vi "Parameter.vi"(9 "In":string, 10 "VIId":string, 11 "VariablesRef":T3) -> ()   [LabVIEW 2018, in "Number.lvlib"]
uses:
  Number.lvlib
  <userlib>/_OpenG.lib/dictionary/dictionary.llb/Dictionary Object RefNum__ogtk.ctl
  <userlib>/_OpenG.lib/dictionary/dictionary.llb/Dictionary Object RefNum - Enum__ogtk.ctl
  <vilib>/addons/_JKI.lib/Serialization/JSON/JKI JSON Serialization.lvlib
panel:
  in  "Tab Control":enum32{"Config", "控件"}(tab)
  in  "ArrayType":T1(tab)
  in  "数值_InitialNumber":dbl caption="数值"
  in  "范围_RandomNumber":dbl=1.0 caption="范围" min=1.0
  in  "变量数量_CalculateNumber":enum16{"Single", "Double"}(ring) caption="变量数量"
  in  "公式":string
  in  "数值X_CalculateNumber":string(combo) caption="数值x"
  in  "数值Y_CalculateNumber":string(combo) caption="数值y"
  in  "数值Y_CompareNumber":string(combo) caption="数值y"
  in  "数值X_CompareNumber":string(combo) caption="数值x"
  in  "比较类型__CompareNumber":u16(ring) caption="比较类型" items=["=", "!=", ">", ">=", "<", "<="]
  in  "方法":T2(ring) caption="方法(Method)"
  # "例：x+1 或 x+y-2"
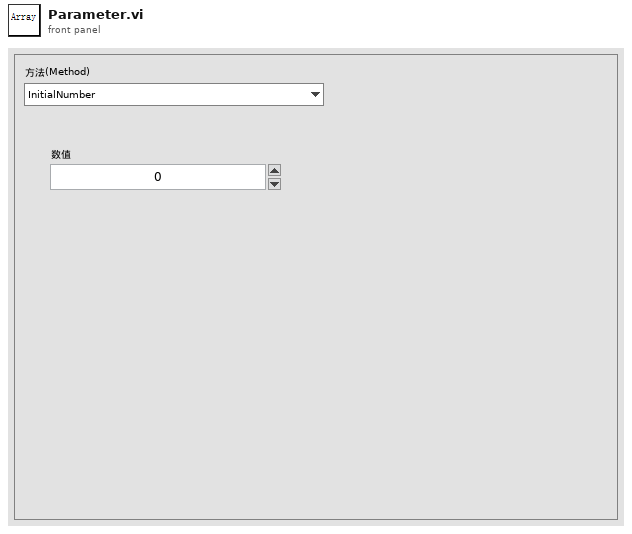
[diagram p1: front panel]
types:
  T1 = enum32{"InitialNumber", "RandomNumber", "CalculateNumber", "CompareNumber"}
  T2 = enum16{"InitialNumber", "RandomNumber", "CalculateNumber", "CompareNumber"}
  T3 = typedef "Dictionary Object RefNum__ogtk.ctl" = refnum<k1>
  T4 = cluster{"InitialNumber":cluster{"json":cluster{"Method":string, "InitialNum":dbl}}, "RandomNumber":cluster{"json":cluster{"Method":string, "Seed":dbl}}, "CalculateNumber":cluster{"json":cluster{"Method":string, "Type":string, "NumxVar":string, "NumyVar":string, "Formula":string}}, "CompareNumber":cluster{"json":cluster{"Method":string, "Type":string, "NumxVar":string, "NumyVar":string}}}
  T5 = enum32{"Invalid", "Standard", "Closed", "Hidden", "Minimized", "Maximized"}
  T6 = enum32{"invalid app kind", "Development System", "Run Time System", "Student Edition", "Embedded LabVIEW", "Evaluation", "Custom"}
  T7 = cluster{"Core":cluster{"Current VI Reference":refnum<vi>, "Close Panel on Exit?":bool}, "Parameter":cluster{"VariableRef":T3}, "Synchronize":cluster{"EnqueueData":cluster{"Action":enum16{"Create", "Query", "Revert", "UpdateVariable", "Close"}, "Data":variant}, "Echo":cluster{"VIRef":refnum<vi>, "JsonOut":string, "Status":string}, "Communicate":cluster{"ID":string, "JsonIn":string, "VarRef":T3}, "Queue":refnum<queue>}, "NumberClusters":cluster{"InitialNumber":cluster{"json":cluster{"Method":string, "InitialNum":dbl}}, "RandomNumber":cluster{"json":cluster{"Method":string, "Seed":dbl}}, "CalculateNumber":cluster{"json":cluster{"Method":string, "Type":string, "NumxVar":string, "NumyVar":string, "Formula":string}}, "CompareNumber":cluster{"json":cluster{"Method":string, "Type":string, "NumxVar":string, "NumyVar":string}}}}
  T8 = cluster{"EnqueueData":cluster{"Action":enum16{"Create", "Query", "Revert", "UpdateVariable", "Close"}, "Data":variant}, "Echo":cluster{"VIRef":refnum<vi>, "JsonOut":string, "Status":string}, "Communicate":cluster{"ID":string, "JsonIn":string, "VarRef":T3}, "Queue":refnum<queue>}
  T9 = cluster{"Current VI Reference":refnum<vi>, "Close Panel on Exit?":bool}
  T10 = cluster{"json":cluster{"Method":string, "InitialNum":dbl}}
  T11 = cluster{"json":cluster{"Method":string, "Seed":dbl}}
  T12 = cluster{"json":cluster{"Method":string, "Type":string, "NumxVar":string, "NumyVar":string, "Formula":string}}
  T13 = cluster{"json":cluster{"Method":string, "Type":string, "NumxVar":string, "NumyVar":string}}
  T14 = cluster{"Action":enum16{"Create", "Query", "Revert", "UpdateVariable", "Close"}, "Data":variant}
  T15 = cluster{"ID":string, "JsonIn":string, "VarRef":T3}
  T16 = enum16{"Create", "Query", "Revert", "UpdateVariable", "Close"}
  T17 = cluster{"VIRef":refnum<vi>, "JsonOut":string, "Status":string}
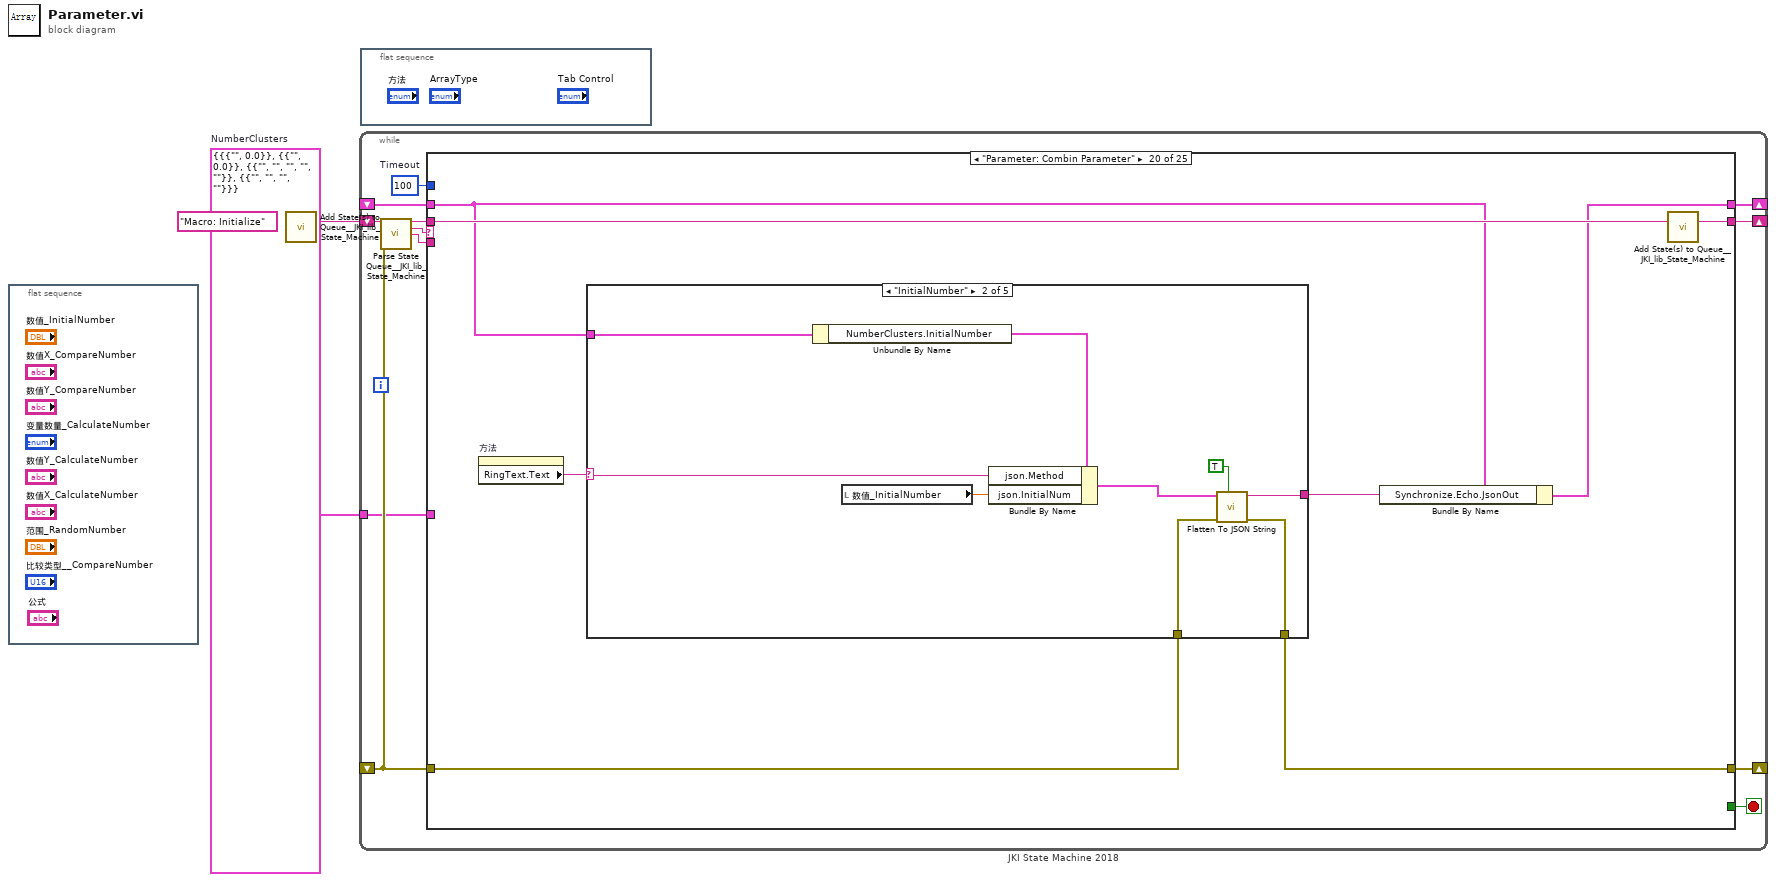
[diagram p0: block diagram]
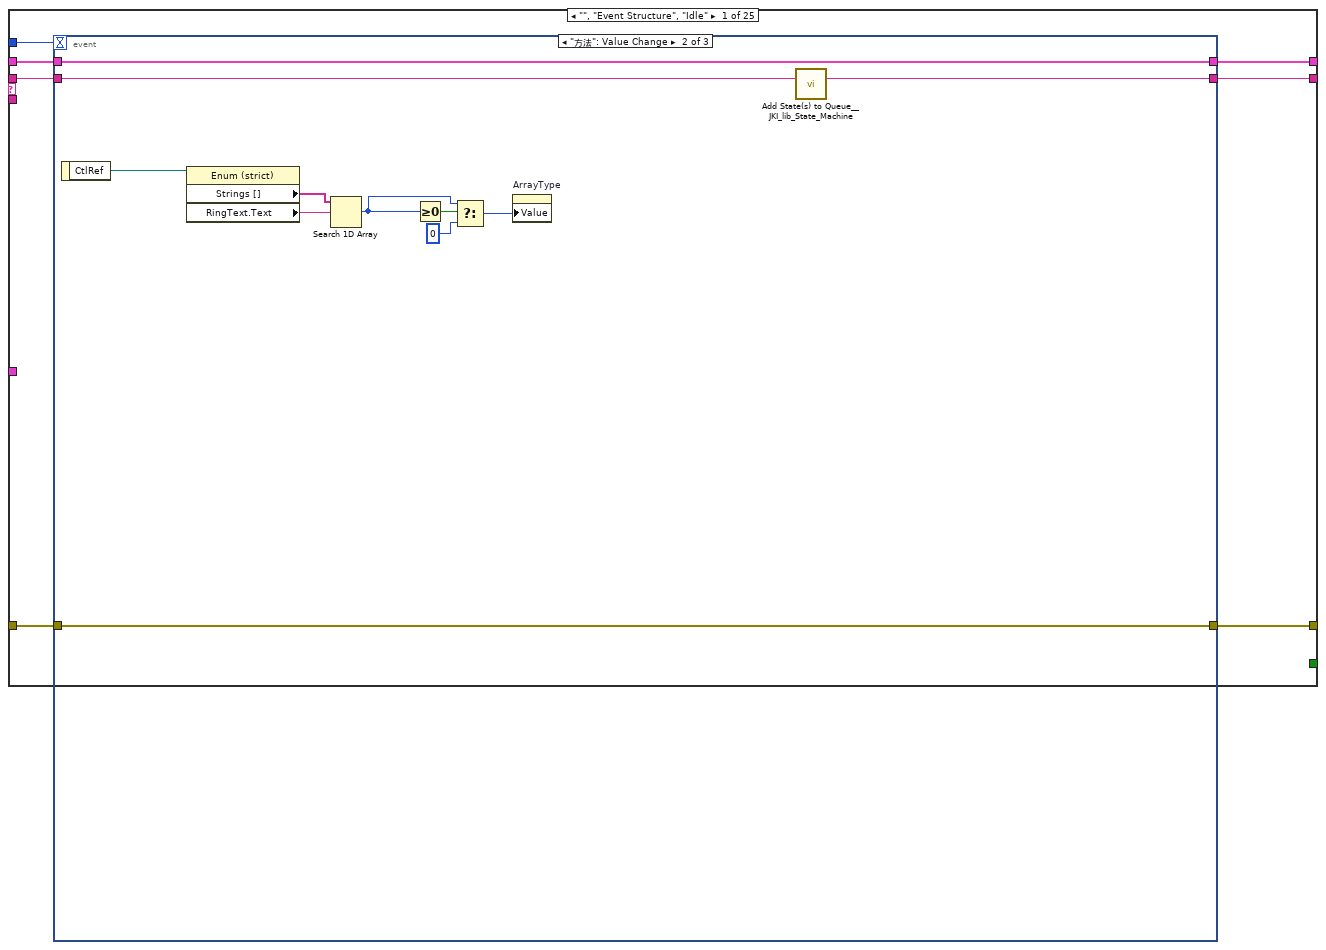
[diagram p2: hidden frame]
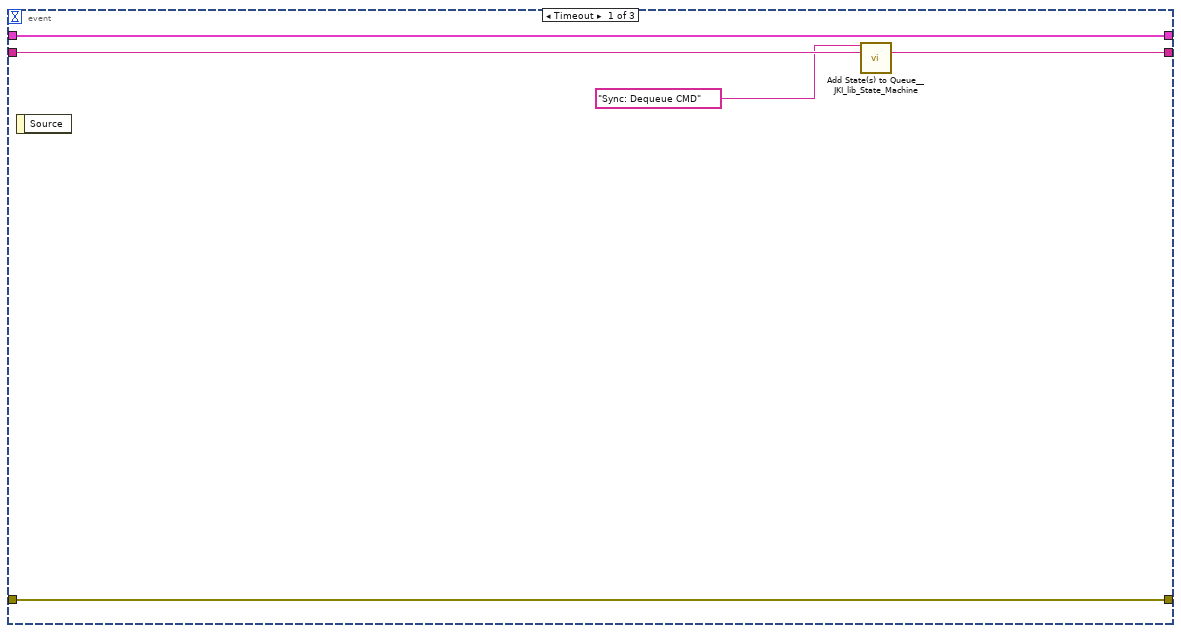
[diagram p3: hidden frame]
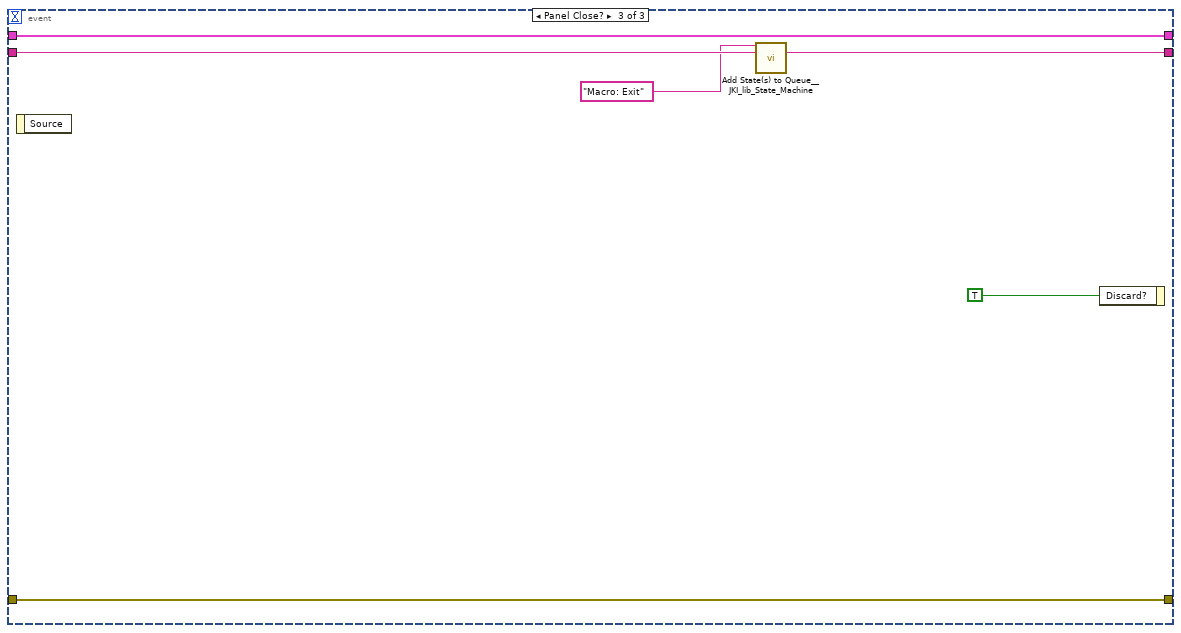
[diagram p4: hidden frame]
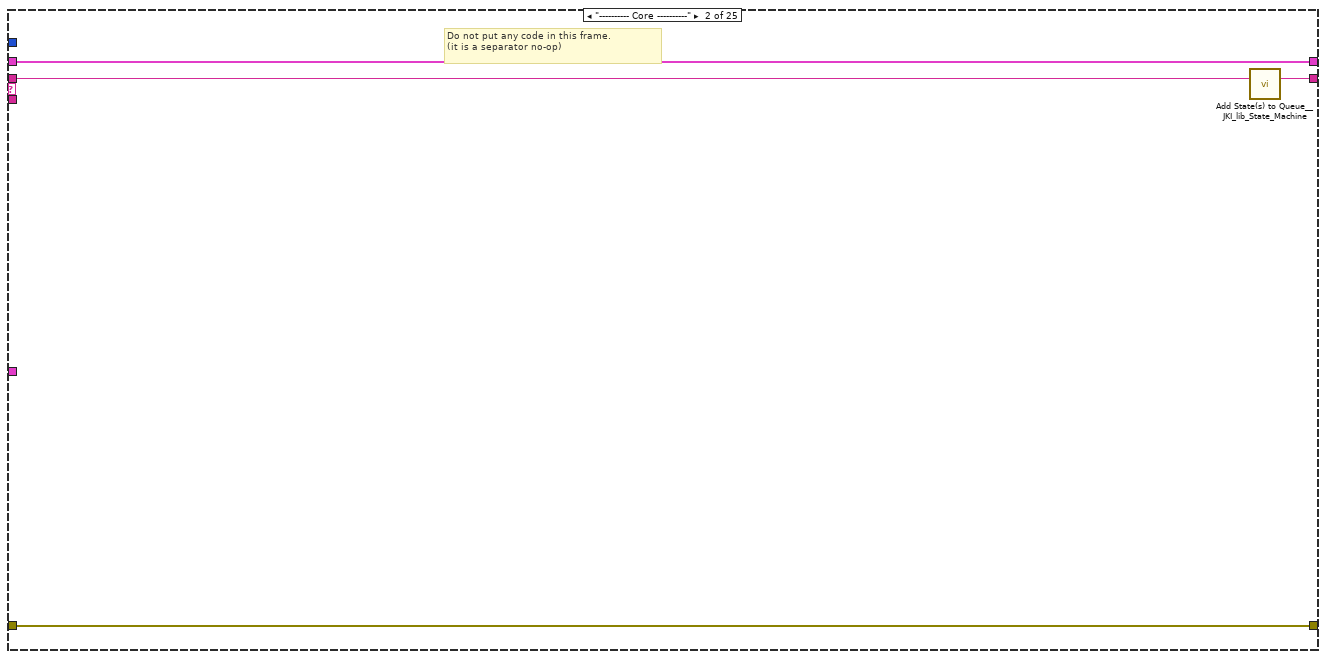
[diagram p5: hidden frame]
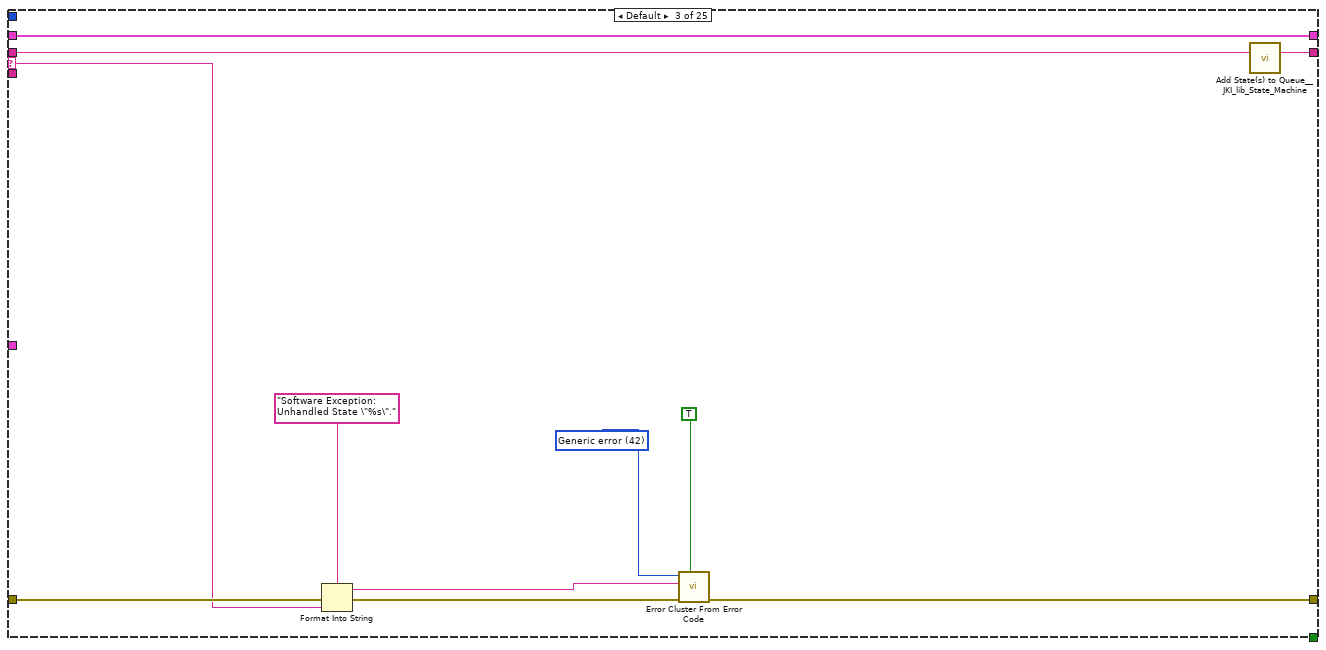
[diagram p6: hidden frame]
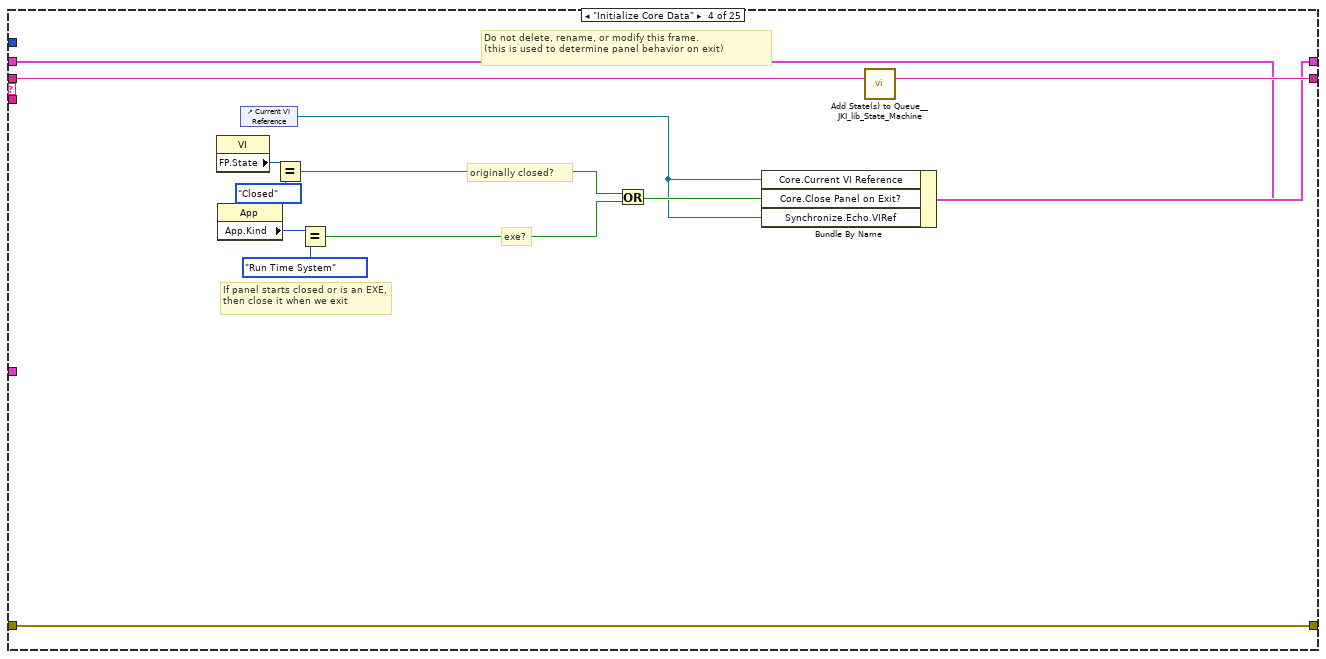
[diagram p7: hidden frame]
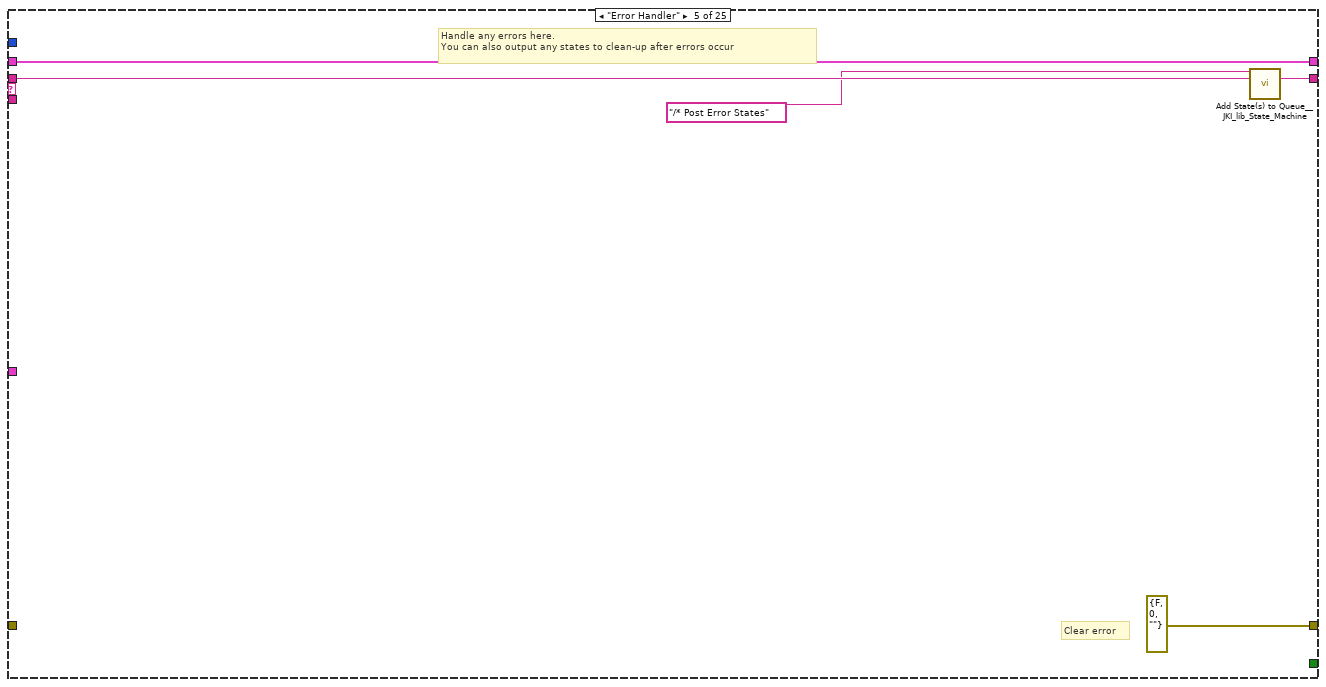
[diagram p8: hidden frame]
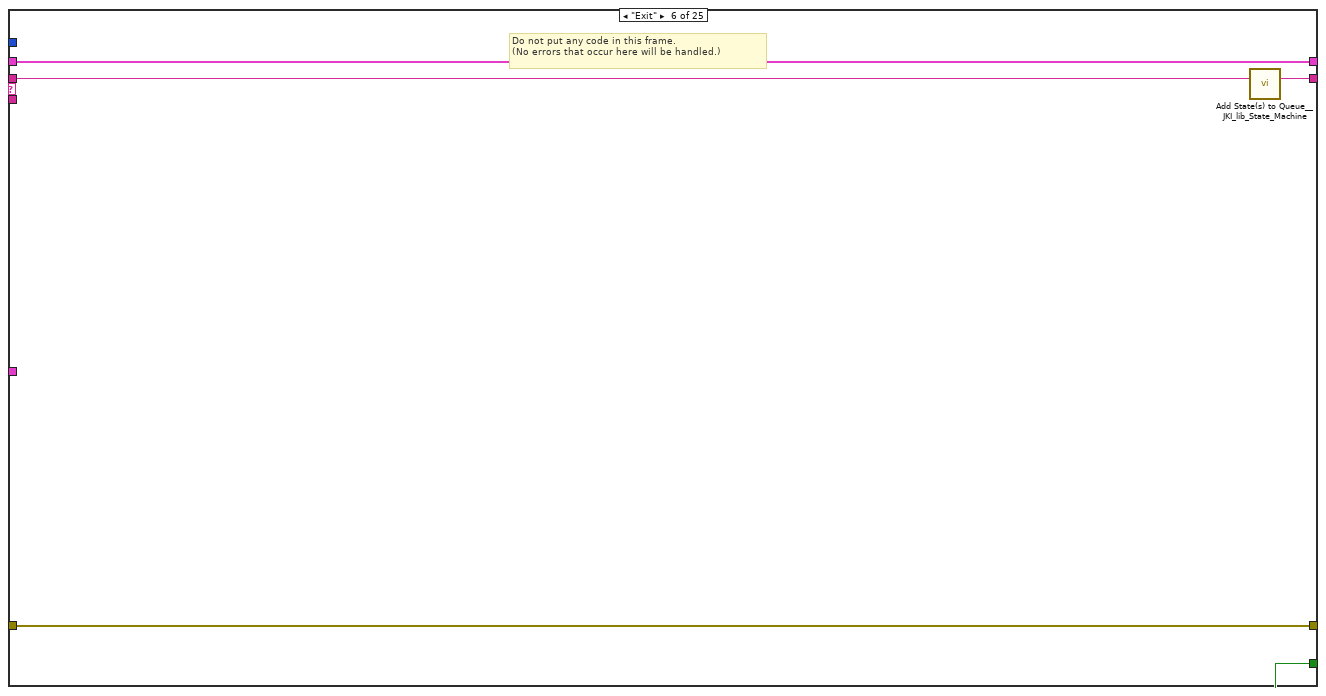
[diagram p9: hidden frame]
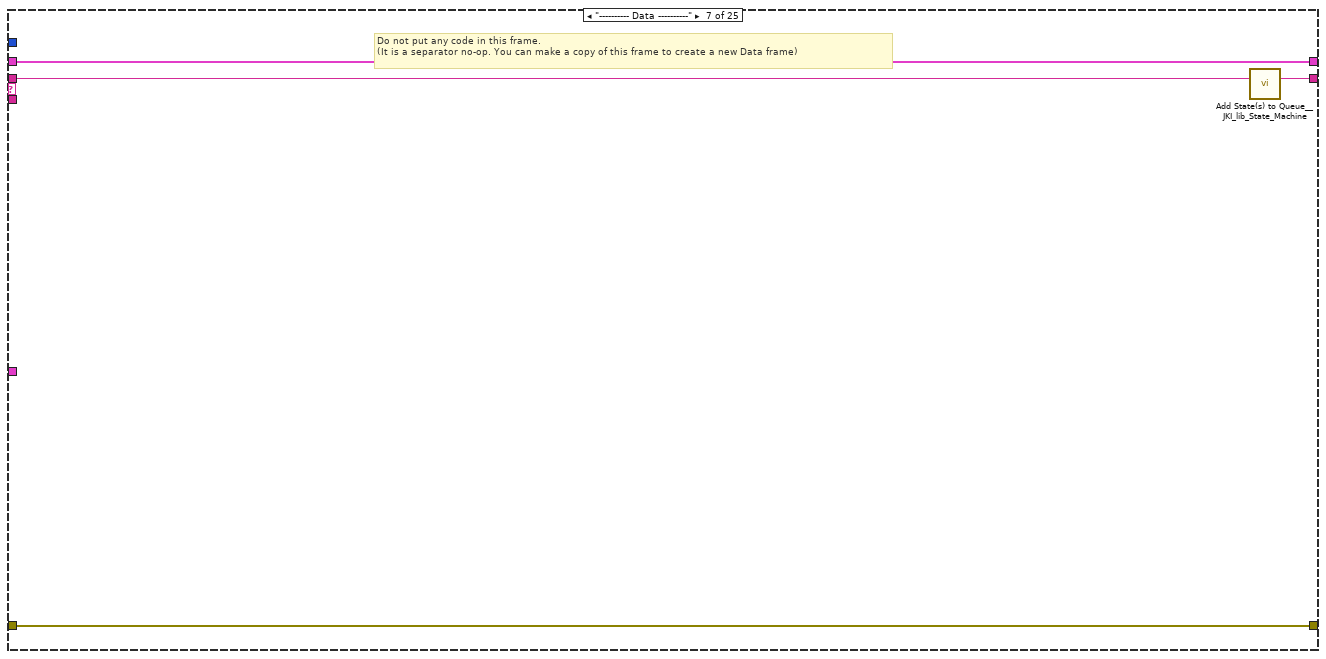
[diagram p10: hidden frame]
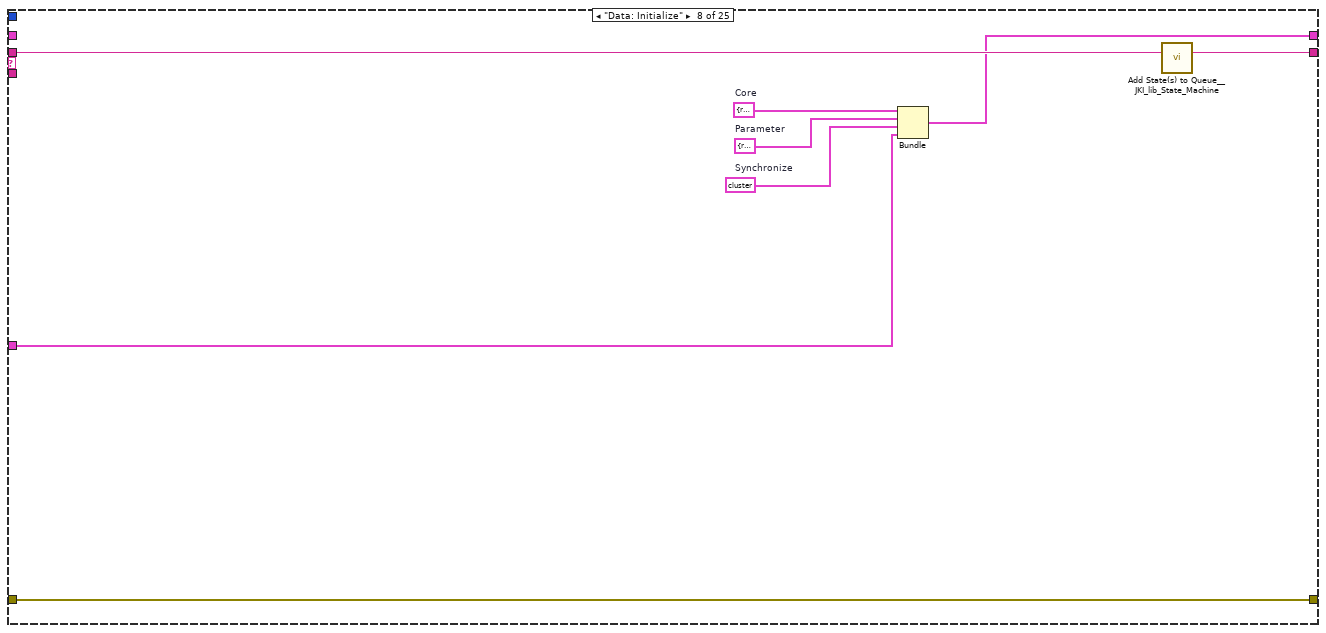
[diagram p11: hidden frame]
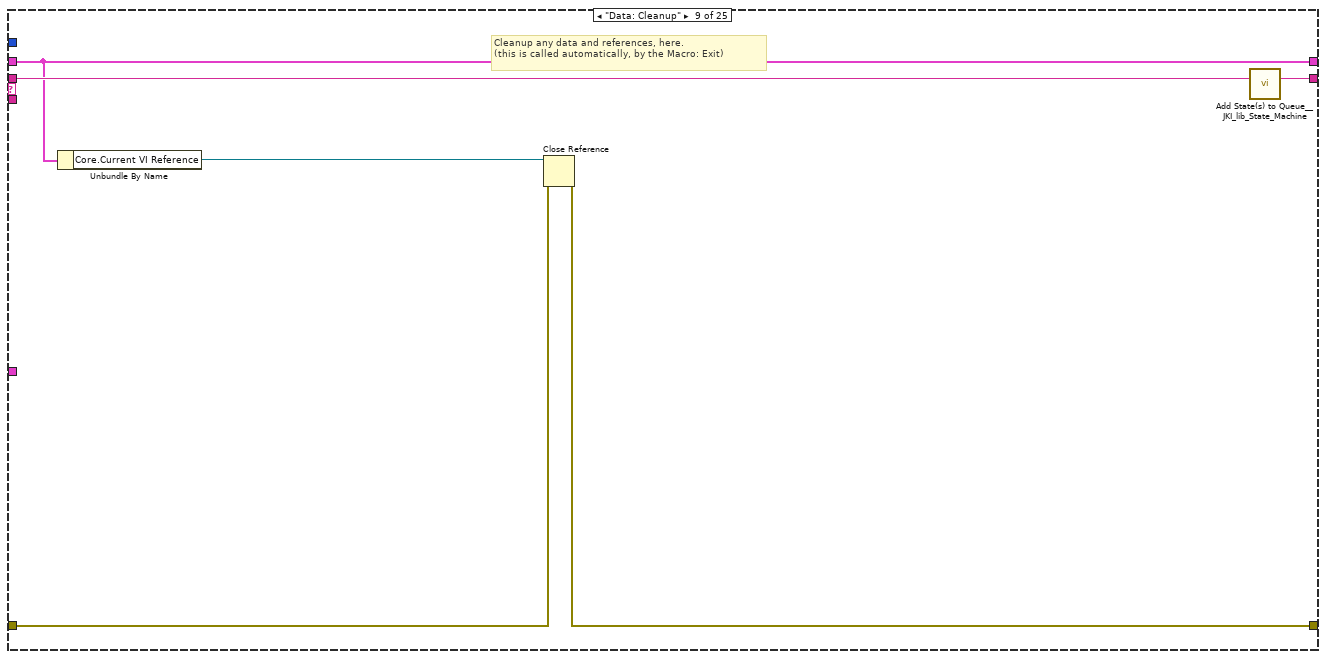
[diagram p12: hidden frame]
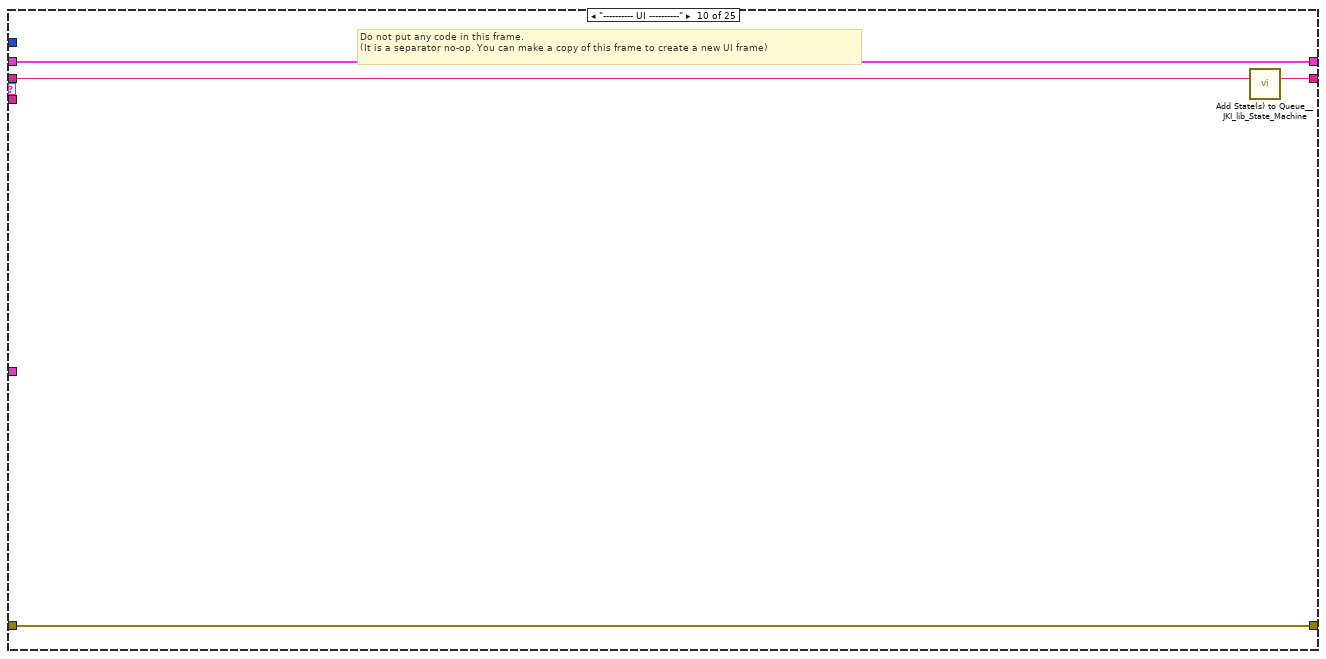
[diagram p13: hidden frame]
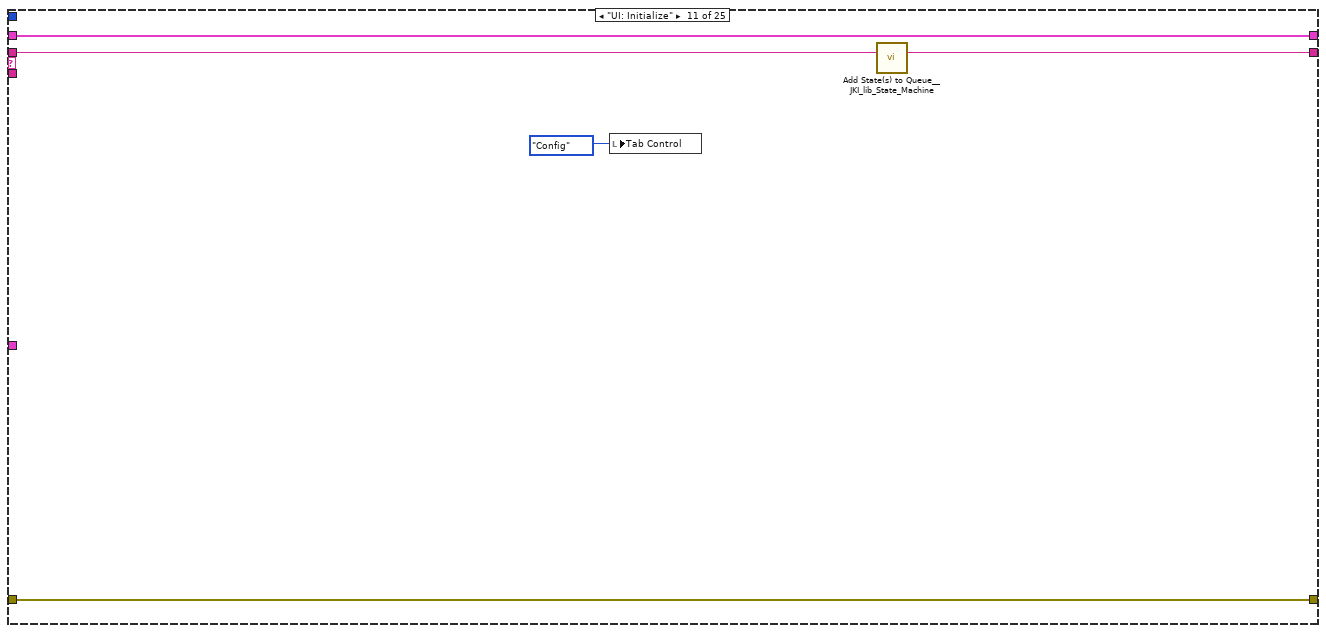
[diagram p14: hidden frame]
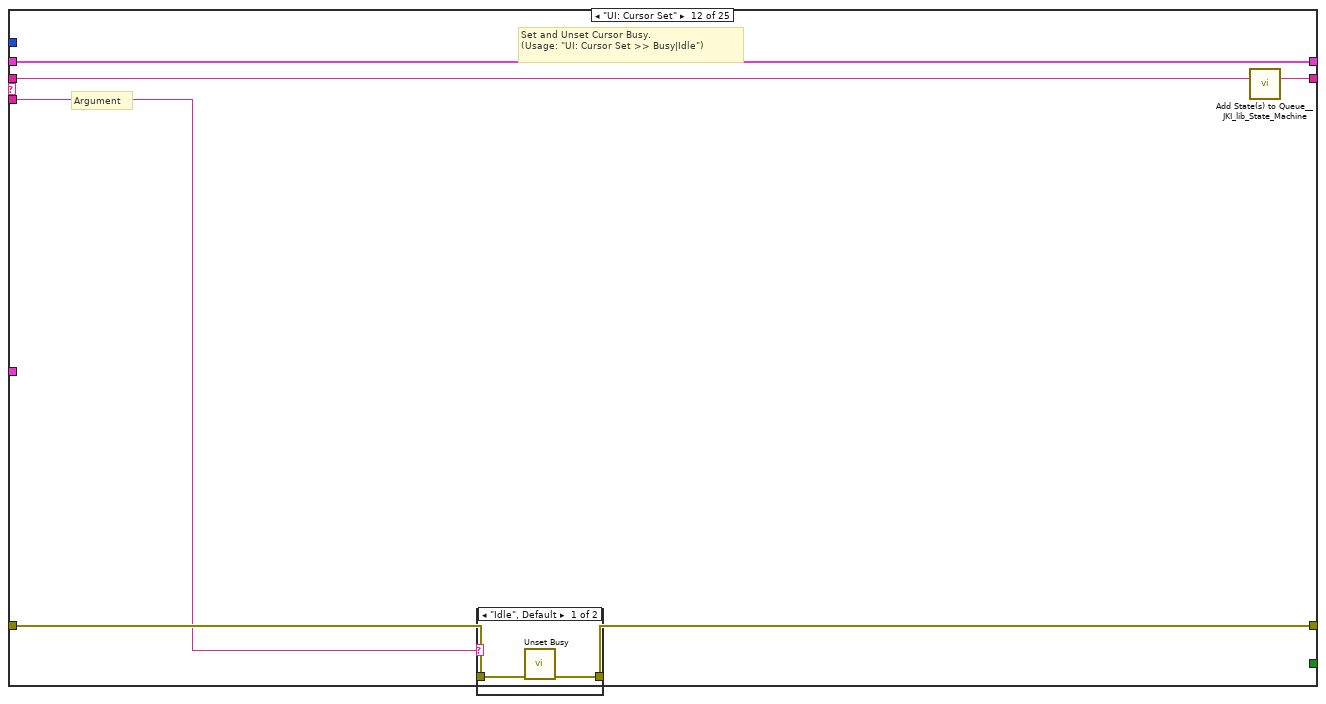
[diagram p15: hidden frame]
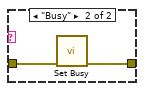
[diagram p16: hidden frame]
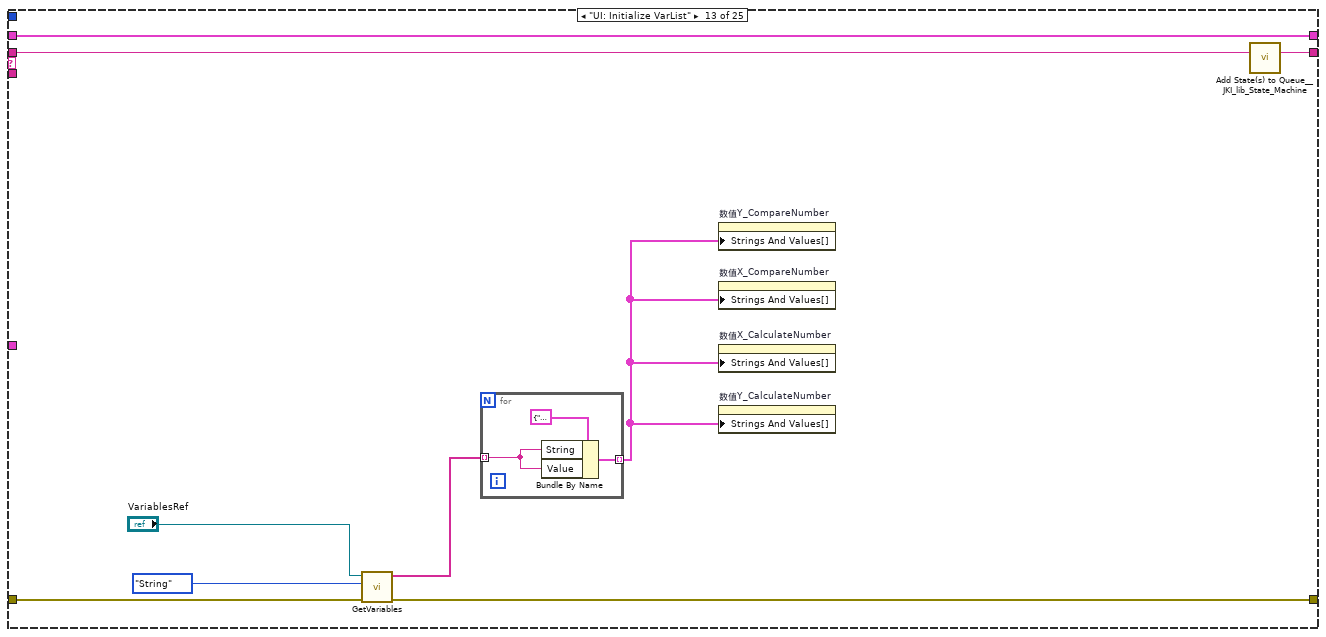
[diagram p17: hidden frame]
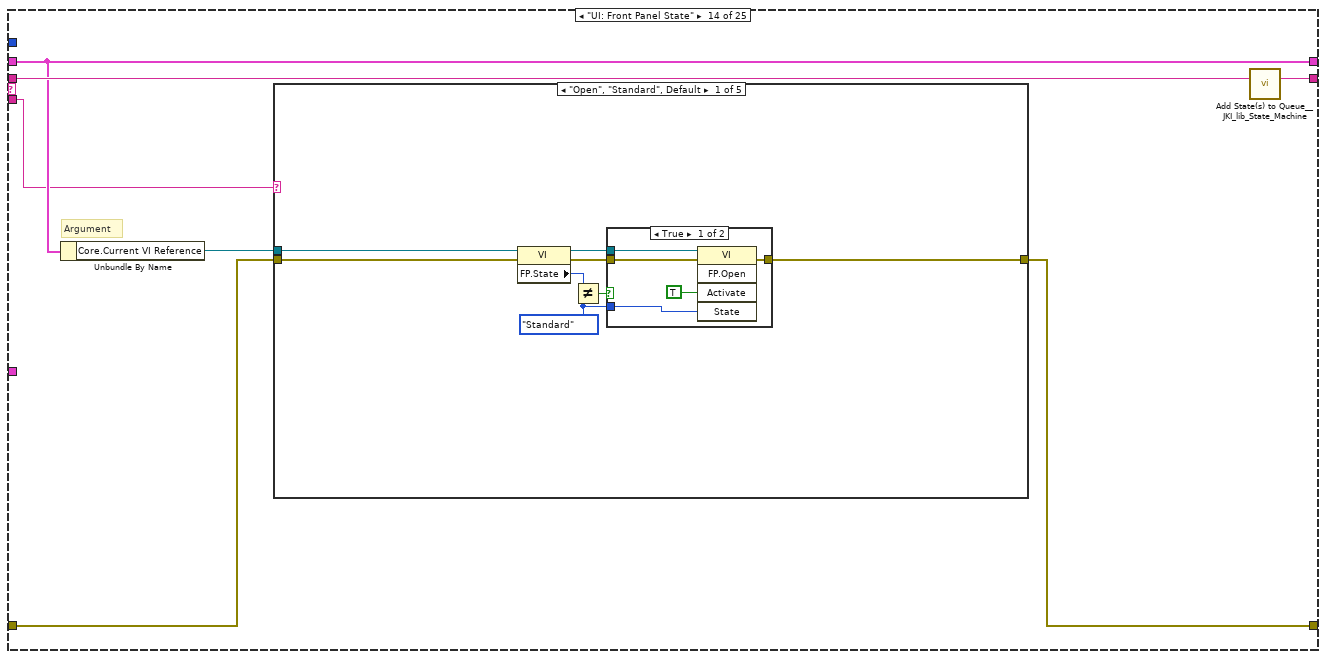
[diagram p18: hidden frame]
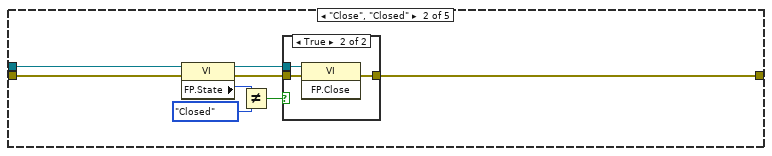
[diagram p20: hidden frame]
diagram:
  w1 = T4 {"InitialNumber"={"json"={"Method"="", "InitialNum"=0.0}}, "RandomNumber"={"json"={"Method"="", "Seed"=0.0}}, "CalculateNumber"={"json"={"Method"="", "Type"="", "NumxVar"="", "NumyVar"="", "Formula"=""}}, "CompareNumber"={"json"={"Method"="", "Type"="", "NumxVar"="", "NumyVar"=""}}}  # NumberClusters
  n1 = flat-sequence {
    frame #0 {
    }
  }
  n2 = call <vilib>:"Add State(s) to Queue__JKI_lib_State_Machine.vi"("State(s) in (\"\")"="Macro: Initialize") -> ("States Out"=w3:string)  [unwired: 14 in]
  n3 = while "JKI State Machine 2018" {
    shift-right: [w8] -> _
    shift-left: _ -> [w7]
    shift-right: [w11] -> _
    shift-left: _ -> [w5]
    shift-right: [w10] -> _
    shift-left: w3 -> [w12]
    tunnel: w1 -> [w4]
    stop <- w9 stop-if-true
    w6 = 100  # Timeout
    n4 = call <vilib>:"Parse State Queue__JKI_lib_State_Machine.vi"("State Queue"=w12, "Error In (no error)"=w5) -> ("Remaining States"=w14:string, "Current State"=w15:string, "Arguments"=w13:string)  [unwired: 11 in]
    n5 = case shown="\"Parameter: Combin Parameter\"" w15 {
      selector: w15 -> [_ _ w49 _ _ _ _ _ _ _ _ _ _ _ _ _ _ _ _ _ _ _ _ _ _]
      tunnel: w14 -> [w22 w48 w53 w72 w77 w82 w86 w94 w100 w104 w109 w115 w128 w138 w207 w212 w222 w226 w234 w313 w359 w368 w383 w427 w442]
      tunnel: w13 -> [_ _ _ _ _ _ _ _ _ _ _ w110 _ w132 _ _ _ _ _ _ _ _ _ _ _]
      tunnel: w7 -> [w20 w45 w51 w65 w74 w80 w83 _ w95 w101 w106 w113 w126 w134 w204 w209 w219 w223 w229 w310 w356 w361 w381 w424 w431]
      tunnel: [w19 w46 w55 w69 errorcluster {"status"=FALSE, "code"=0, "source"=""} ("error out") w79 w84 w92 w96 w102 w105 w111 w125 w135 w205 w210 w220 w224 w230 w309 w357 w365 w370 w422 w429] -> w11
      tunnel: w5 -> [w18 w46 w54 w69 _ w79 w84 w92 w97 w102 w105 w112 w123 w136 w205 w210 w220 w224 w231 w308 w357 w366 w379 w423 w430]
      tunnel: [w21 w47 w52 w71 w76 w81 w85 w93 w99 w103 w108 w114 w127 w137 w206 w211 w221 w225 w233 w312 w358 w367 w382 w426 w441] -> w10
      tunnel: [_ _ _ _ _ TRUE _ _ _ _ _ _ _ _ _ _ _ _ _ _ _ _ _ _ _] -> w9
      tunnel: [w17 w45 w51 w70 w74 w80 w83 w89 w95 w101 w106 w113 w126 w134 w204 w209 w219 w223 w229 w311 w356 w363 w372 w424 w431] -> w8
      tunnel: w6 -> [w16 _ _ _ _ _ _ _ _ _ _ _ _ _ _ _ _ _ _ _ _ _ _ _ _]
      tunnel: w4 -> [_ _ _ _ _ _ _ w87 _ _ _ _ _ _ _ _ _ _ _ _ _ _ _ _ _]
      frame "", "Event Structure", "Idle" {
        n6 = event shown="[1] \"方法\": Value Change" {
          selector: _ -> [_ _ _]
          dyn-events: _ -> [_ _ _]
          timeout: w16 -> [_ _ _]
          tunnel: w22 -> [w27 w38 w44]
          tunnel: [w26 w37 w43] -> w21
          tunnel: w20 -> [w24 w35 w41]
          tunnel: [w25 w36 w42] -> w19
          tunnel: w18 -> [w25 w36 w42]
          tunnel: [w24 w35 w41] -> w17
          event Timeout {
            n7 = event-data() -> ()  [unwired: 1 in, 1 out]
            n8 = call <vilib>:"Add State(s) to Queue__JKI_lib_State_Machine.vi"("State(s) in Front (\"\")"="Sync: Dequeue CMD" ("State(s) in Front (\"\")"), "State(s) in (\"\")"=w27) -> ("States Out"=w26:string)  [unwired: 13 in]
          }
          event "方法": Value Change {
            n9 = event-data() -> ("CtlRef"=w31:refnum<vi>)  [unwired: 1 in]
            n10 = property class="Enum (strict)"(reference=w31) -> ("Strings []"=w30:string[], "RingText.Text"=w29:string)  [unwired: 1 in, 2 out]
            n11 = Search 1D Array(1D array=w30, element=w29) -> (index of element=w33:i32)  [unwired: 1 in]
            n12 = Greater Or Equal To 0?(x=w33) -> (x >= 0?=w34:bool)
            n13 = Select(t=w33, s=w34, f=0) -> (s? t:f=w28:i32)
            n14 = property on="ArrayType" class="TabCtl (strict)"("Value"=w28) -> ()  [unwired: 2 in, 2 out]
            n15 = call <vilib>:"Add State(s) to Queue__JKI_lib_State_Machine.vi"("State(s) in (\"\")"=w38) -> ("States Out"=w37:string)  [unwired: 14 in]
          }
          event Panel Close? {
            n16 = event-data() -> ()  [unwired: 1 in, 1 out]
            n17 = call <vilib>:"Add State(s) to Queue__JKI_lib_State_Machine.vi"("State(s) in Front (\"\")"="Macro: Exit", "State(s) in (\"\")"=w44) -> ("States Out"=w43:string)  [unwired: 13 in]
            n18 = event-data("Discard?"=TRUE) -> ()  [unwired: 1 in, 1 out]
          }
        }
      }
      frame "---------- Core ----------" {
        # "Do not put any code in this frame.\n(it is a separator no-op)"
        n19 = call <vilib>:"Add State(s) to Queue__JKI_lib_State_Machine.vi"("State(s) in (\"\")"=w48) -> ("States Out"=w47:string)  [unwired: 14 in]
      }
      frame Default {
        w58 = 42 items=["No error", "Argument error", "Memory is full", "Out of zone", "End of file", "File already open", "Generic file I/O error", "File not found", "File permission error", "Disk is full", "Duplicate path", "Too many files open", "System feature not enabled", "Resource file not found", "Cannot add resource", "Resource not found", "Image not found", "Image memory error", "Pen does not exist", "Config type invalid", "Config token not found", "Config parse error", "Config memory error", "Bad external code format", "Bad external code offset", "External code not present", "Null window", "Destroy window error", "Null menu", "Print aborted", "Bad print record", "Print driver error", "Windows error during printing", "Memory error during printing", "Print dialog error", "Generic print error", "Invalid device refnum", "Device not found", "Device parameter error", "Device unit error", "Cannot open device", "Device call aborted", "Generic error", "Cancelled by user", "Object ID too low", "Object ID too high", "Object not in heap", "Unknown heap", "Unknown object (invalid DefProc)", "Unknown object (DefProc not in table)", "Message out of range", "Invalid (null) method", "Unknown message", "Manager call not supported", "Bad address", "Network operation in progress", "Network operation timed out", "Connection is busy", "Network attribute not supported", "Network error", "Address in use", "System out of memory", "Connection aborted", "Connection refused", "Not connected", "Already connected", "Connection closed", "Initialization error (interapplication manager)", "Bad occurrence", "Wait on unbound occurrence handler", "Occurrence queue overflow", "Datalog type conflict", "Unused", "Unrecognized type (interapplication manager)", "Memory corrupt", "Failed to make temporary DLL", "Old CIN version", "Drag socket not found", "Failed to load drop-object", "Failed to register OLE object", "Failed to release OLE object", "Format specifier type mismatch", "Unknown format specifier", "Too few format specifiers", "Too many format specifiers", "Scan failed", "Newer CIN version", "Error converting to variant", "Runtime menu error", "Password tampered", "Variant attribute not found", "Incompatible variant data type", "Event data is not available", "Event Store is not present", "Occurrence is not found", "Event Queue is not created", "Event info is not available", "Refnum passed is NULL", "Error retrieving Class GUID", "Error retrieving CoClass GUID", "Error retrieving TypeLib GUID.", "Bad built application magic bytes.", "Specific driver is different from the specific driver associated with the Logical Name.", "There is no session opened to the class driver.", "Max Error", "MAX - Error with config objects", "MAX - Error loading configuration", "MAX - Group not supported"]
        n20 = Format Into String(format string="Software Exception: Unhandled State \"%s\"." ("message"), error in=w54, w49) -> (resulting string=w57:string, error out=w56:errorcluster)  [unwired: 1 in]
        n21 = call <vilib>:"Error Cluster From Error Code.vi"("show call chain? (False)"=TRUE, "error in (no error)"=w56, "error message (\"\")"=w57, "error code (0)"=w58) -> ("error out"=w55:errorcluster)  [unwired: 5 in]
        n22 = call <vilib>:"Add State(s) to Queue__JKI_lib_State_Machine.vi"("State(s) in (\"\")"=w53) -> ("States Out"=w52:string)  [unwired: 14 in]
      }
      frame "Initialize Core Data" {
        # "Do not delete, rename, or modify this frame.\n(this is used to determine panel behavior on exit)"
        # "originally closed?"
        # "exe?"
        # "If panel starts closed or is an EXE, then close it when we exit"
        n23 = property class="VI"() -> ("FP.State"=w63:T5)  [unwired: 2 in, 2 out]
        n24 = property class="App"() -> ("App.Kind"=w68:T6)  [unwired: 2 in, 2 out]
        n25 = control-ref of="Current VI Reference"() -> (w60:refnum<vi>)
        n26 = Equal?(x=w63, y=T5."Closed" ("Front Panel Window:State")) -> (x = y?=w61:bool)
        n27 = Equal?(x=w68, y=T6."Run Time System" ("Application:Kind")) -> (x = y?=w66:bool)
        n28 = Or(x=w61, y=w66) -> (x .or. y?=w64:bool)
        n29 = Bundle By Name(cluster=w65, "Core.Current VI Reference"=w60, "Core.Close Panel on Exit?"=w64, "Synchronize.Echo.VIRef"=w60) -> (w70:T7)
        n30 = call <vilib>:"Add State(s) to Queue__JKI_lib_State_Machine.vi"("State(s) in (\"\")"=w72) -> ("States Out"=w71:string)  [unwired: 14 in]
      }
      frame "Error Handler" {
        # "Handle any errors here.\nYou can also output any states to clean-up after errors occur"
        # "Clear error"
        n31 = call <vilib>:"Add State(s) to Queue__JKI_lib_State_Machine.vi"("State(s) in Front (\"\")"="/* Post Error States", "State(s) in (\"\")"=w77) -> ("States Out"=w76:string)  [unwired: 13 in]
      }
      frame "Exit" {
        # "Do not put any code in this frame.\n(No errors that occur here will be handled.)"
        n32 = call <vilib>:"Add State(s) to Queue__JKI_lib_State_Machine.vi"("State(s) in (\"\")"=w82) -> ("States Out"=w81:string)  [unwired: 14 in]
      }
      frame "---------- Data ----------" {
        # "Do not put any code in this frame.\n(It is a separator no-op. You can make a copy of this frame to create a new Data frame)"
        n33 = call <vilib>:"Add State(s) to Queue__JKI_lib_State_Machine.vi"("State(s) in (\"\")"=w86) -> ("States Out"=w85:string)  [unwired: 14 in]
      }
      frame "Data: Initialize" {
        w88 = cluster{"VariableRef":T3} {"VariableRef"=refnum}  # Parameter
        w90 = T8 {"EnqueueData"={"Action"=enum."Create", "Data"=variant}, "Echo"={"VIRef"=refnum, "JsonOut"="", "Status"=""}, "Communicate"={"ID"="", "JsonIn"="", "VarRef"=refnum}, "Queue"=refnum}  # Synchronize
        w91 = T9 {"Current VI Reference"=refnum, "Close Panel on Exit?"=FALSE}  # Core
        n34 = Bundle("Core"=w91, "Parameter"=w88, "Synchronize"=w90, "NumberClusters"=w87) -> (w89:T7)  [unwired: 1 in]
        n35 = call <vilib>:"Add State(s) to Queue__JKI_lib_State_Machine.vi"("State(s) in (\"\")"=w94) -> ("States Out"=w93:string)  [unwired: 14 in]
      }
      frame "Data: Cleanup" {
        # "Cleanup any data and references, here.\n(this is called automatically, by the Macro: Exit)"
        n36 = Unbundle By Name(w95) -> ("Core.Current VI Reference"=w98:refnum<vi>)
        n37 = Close Reference(reference=w98, error in (no error)=w97) -> (error out=w96:errorcluster)
        n38 = call <vilib>:"Add State(s) to Queue__JKI_lib_State_Machine.vi"("State(s) in (\"\")"=w100) -> ("States Out"=w99:string)  [unwired: 14 in]
      }
      frame "---------- UI ----------" {
        # "Do not put any code in this frame.\n(It is a separator no-op. You can make a copy of this frame to create a new UI frame)"
        n39 = call <vilib>:"Add State(s) to Queue__JKI_lib_State_Machine.vi"("State(s) in (\"\")"=w104) -> ("States Out"=w103:string)  [unwired: 14 in]
      }
      frame "UI: Initialize" {
        n40 = local write "Tab Control"(enum32{"Config", "控件"}."Config" ("Tab Control")) -> ()
        n41 = call <vilib>:"Add State(s) to Queue__JKI_lib_State_Machine.vi"("State(s) in (\"\")"=w109) -> ("States Out"=w108:string)  [unwired: 14 in]
      }
      frame "UI: Cursor Set" {
        # "Argument"
        # "Set and Unset Cursor Busy.\n(Usage: \"UI: Cursor Set >> Busy|Idle\")"
        n42 = case shown="\"Idle\", Default" w110 {
          tunnel: w112 -> [w117 w119]
          tunnel: [w116 w118] -> w111
          frame "Idle", Default {
            n43 = call <vilib>:"Unset Busy.vi"("error in (no error)"=w117) -> ("error out"=w116:errorcluster)  [unwired: 10 in]
          }
          frame "Busy" {
            n44 = call <vilib>:"Set Busy.vi"("error in (no error)"=w119) -> ("error out"=w118:errorcluster)  [unwired: 9 in, 1 out]
          }
        }
        n45 = call <vilib>:"Add State(s) to Queue__JKI_lib_State_Machine.vi"("State(s) in (\"\")"=w115) -> ("States Out"=w114:string)  [unwired: 14 in]
      }
      frame "UI: Initialize VarList" {
        n46 = call "GetVariables.vi"("error in (no error)"=w123, "VariableType"=enum16{"String", "StringArray"}."String", "DicRef"="VariablesRef") -> ("error out"=w125:errorcluster, "VariableArray"=w121:string[])  [unwired: 7 in]
        n47 = for {
          tunnel: w121 -> [w129] mode=indexing
          tunnel: [w130] -> w120 mode=indexing
          n48 = Bundle By Name(cluster=cluster{"String":string, "Value":string} {"String"="", "Value"=""}, "String"=w129, "Value"=w129) -> (w130:cluster{"String":string, "Value":string})
        }
        n49 = property on="数值Y_CompareNumber" class="CmbBox"("Strings And Values[]"=w120) -> ()  [unwired: 2 in, 2 out]
        n50 = property on="数值X_CompareNumber" class="CmbBox"("Strings And Values[]"=w120) -> ()  [unwired: 2 in, 2 out]
        n51 = property on="数值X_CalculateNumber" class="CmbBox"("Strings And Values[]"=w120) -> ()  [unwired: 2 in, 2 out]
        n52 = property on="数值Y_CalculateNumber" class="CmbBox"("Strings And Values[]"=w120) -> ()  [unwired: 2 in, 2 out]
        n53 = call <vilib>:"Add State(s) to Queue__JKI_lib_State_Machine.vi"("State(s) in (\"\")"=w128) -> ("States Out"=w127:string)  [unwired: 14 in]
      }
      frame "UI: Front Panel State" {
        # "Argument"
        n54 = Unbundle By Name(w134) -> ("Core.Current VI Reference"=w133:refnum<vi>)
        n55 = case shown="\"Open\", \"Standard\", Default" w132 {
          tunnel: w136 -> [w144 w159 w170 w183 w196]
          tunnel: [w146 w160 w172 w185 w198] -> w135
          tunnel: w133 -> [w145 w157 w171 w184 w197]
          frame "Open", "Standard", Default {
            w139 = T5."Standard" ("State")
            n56 = property class="VI"(reference=w145, error in=w144) -> (reference out=w142:refnum<vi>, error out=w143:errorcluster, "FP.State"=w141:T5)
            n57 = Not Equal?(x=w141, y=w139) -> (x != y?=w140:bool)
            n58 = case shown="True" w140 {
              tunnel: [w150 w152] -> w146
              tunnel: w143 -> [w149 w152]
              tunnel: w142 -> [w148 _]
              tunnel: w139 -> [w147 _]
              frame True {
                n59 = invoke class="VI" method="FP.Open"(reference=w148, error in=w149, "Activate"=TRUE, "State"=w147) -> (error out=w150:errorcluster)  [unwired: 1 in, 4 out]
              }
              frame False {
              }
            }
          }
          frame "Close", "Closed" {
            n60 = property class="VI"(reference=w157, error in=w159) -> (reference out=w156:refnum<vi>, error out=w158:errorcluster, "FP.State"=w154:T5)
            n61 = Not Equal?(x=w154, y=T5."Closed" ("Front Panel Window:State")) -> (x != y?=w153:bool)
            n62 = case shown="True" w153 {
              tunnel: [w161 w164] -> w160
              tunnel: w158 -> [w161 w163]
              tunnel: w156 -> [_ w162]
              frame False {
              }
              frame True {
                n63 = invoke class="VI" method="FP.Close"(reference=w162, error in=w163) -> (error out=w164:errorcluster)  [unwired: 1 in, 2 out]
              }
            }
          }
          frame "Hidden", "Hide" {
            w165 = T5."Hidden" ("State")
            n64 = property class="VI"(reference=w171, error in=w170) -> (reference out=w168:refnum<vi>, error out=w169:errorcluster, "FP.State"=w167:T5)
            n65 = Not Equal?(x=w167, y=w165) -> (x != y?=w166:bool)
            n66 = case shown="True" w166 {
              tunnel: [w176 w177] -> w172
              tunnel: w169 -> [w175 w177]
              tunnel: w168 -> [w174 _]
              tunnel: w165 -> [w173 _]
              frame True {
                n67 = invoke class="VI" method="FP.Open"(reference=w174, error in=w175, "State"=w173) -> (error out=w176:errorcluster)  [unwired: 2 in, 4 out]
              }
              frame False {
              }
            }
          }
          frame "Minimize", "Minimized" {
            w178 = T5."Minimized" ("State")
            n68 = property class="VI"(reference=w184, error in=w183) -> (reference out=w181:refnum<vi>, error out=w182:errorcluster, "FP.State"=w180:T5)
            n69 = Not Equal?(x=w180, y=w178) -> (x != y?=w179:bool)
            n70 = case shown="True" w179 {
              tunnel: [w189 w190] -> w185
              tunnel: w182 -> [w188 w190]
              tunnel: w181 -> [w187 _]
              tunnel: w178 -> [w186 _]
              frame True {
                n71 = invoke class="VI" method="FP.Open"(reference=w187, error in=w188, "State"=w186) -> (error out=w189:errorcluster)  [unwired: 2 in, 4 out]
              }
              frame False {
              }
            }
          }
          frame "Maximize", "Maximized" {
            w191 = T5."Maximized" ("State")
            n72 = property class="VI"(reference=w197, error in=w196) -> (reference out=w194:refnum<vi>, error out=w195:errorcluster, "FP.State"=w193:T5)
            n73 = Not Equal?(x=w193, y=w191) -> (x != y?=w192:bool)
            n74 = case shown="True" w192 {
              tunnel: [w202 w203] -> w198
              tunnel: w195 -> [w201 w203]
              tunnel: w194 -> [w200 _]
              tunnel: w191 -> [w199 _]
              frame True {
                n75 = invoke class="VI" method="FP.Open"(reference=w200, error in=w201, "State"=w199) -> (error out=w202:errorcluster)  [unwired: 2 in, 4 out]
              }
              frame False {
              }
            }
          }
        }
        n76 = call <vilib>:"Add State(s) to Queue__JKI_lib_State_Machine.vi"("State(s) in (\"\")"=w138) -> ("States Out"=w137:string)  [unwired: 14 in]
      }
      frame "---------- Macro ----------" {
        n77 = call <vilib>:"Add State(s) to Queue__JKI_lib_State_Machine.vi"("State(s) in (\"\")"=w207) -> ("States Out"=w206:string)  [unwired: 14 in]
      }
      frame "Macro: Initialize" {
        n78 = call <vilib>:"Add State(s) to Queue__JKI_lib_State_Machine.vi"("State(s) in Front (\"\")"="Data: Initialize\nInitialize Core Data\nUI: Initialize\nSync: Obtain CMD Queue\nSync: Dequeue CMD\nUI: Initialize VarList\nParameter: Parse Parameter", "State(s) in (\"\")"=w212) -> ("States Out"=w211:string)  [unwired: 13 in]
      }
      frame "Macro: Exit" {
        n79 = Unbundle By Name(w219) -> ("Core.Close Panel on Exit?"=w218:bool)
        n80 = Select(t="UI: Front Panel State >> Close", s=w218, f="") -> (s? t:f=w215:string)
        n81 = call <vilib>:"Add State(s) to Queue__JKI_lib_State_Machine.vi"("State(s) in (\"\")"=w215, "State(s) at Back (\"\")"="Sync: Release CMD Queue\nData: Cleanup\nExit") -> ("States Out"=w213:string)  [unwired: 13 in]
        n82 = call <vilib>:"Add State(s) to Queue__JKI_lib_State_Machine.vi"("State(s) in Front (\"\")"=w213, "State(s) in (\"\")"=w222) -> ("States Out"=w221:string)  [unwired: 13 in]
      }
      frame "---------- Parameter ----------" {
        # "Template Separator\n(You can make a copy of, or modify, this frame)"
        n83 = call <vilib>:"Add State(s) to Queue__JKI_lib_State_Machine.vi"("State(s) in (\"\")"=w226) -> ("States Out"=w225:string)  [unwired: 14 in]
      }
      frame "Parameter: Parse Parameter" {
        n84 = Unbundle By Name(w229) -> ("NumberClusters"=w228:T4)
        n85 = Empty String/Path?(string/path="In") -> (empty?=w232:bool)
        n86 = case shown="False" w232 {
          tunnel: "In" -> [w243 _]
          tunnel: w231 -> [w248 w305]
          tunnel: [w247 w305] -> w230
          tunnel: w228 -> [w246 _]
          frame False {
            n87 = Match Pattern(string=w243, regular expression="\"Method\":\"") -> (after substring=w242:string)  [unwired: 1 in, 3 out]
            n88 = Match Pattern(string=w242, regular expression="\",") -> (before substring=w241:string)  [unwired: 1 in, 3 out]
            n89 = case shown="\"CompareNumber\"" w241 {
              tunnel: w243 -> [w256 w266 w284 w301 _]
              tunnel: w248 -> [w254 w264 w282 w299 w304]
              tunnel: [w253 w263 w281 w298 w304] -> w247
              tunnel: w246 -> [w251 w261 w279 w296 _]
              tunnel: [w252 w262 w280 w297 _] -> w236
              frame "InitialNumber" {
                n90 = Unbundle By Name(w251) -> ("InitialNumber"=w250:T10)
                n91 = call <vilib>:"Unflatten From JSON String.vi"("Type and Defaults"=w250, "error in (no error)"=w254, "JSON String"=w256) -> ("error out"=w257:errorcluster, "Variant"=w258:variant)  [unwired: 7 in]
                n92 = Variant To Data(error in=w257, type=w250, Variant=w258) -> (data=w255:T10, error out=w253:errorcluster)
                n93 = Unbundle By Name(w255) -> ("json.Method"=w252:string, "json.InitialNum"=w249:dbl)
                n94 = local write "数值_InitialNumber"(w249) -> ()
              }
              frame "RandomNumber" {
                n95 = Unbundle By Name(w261) -> ("RandomNumber"=w260:T11)
                n96 = call <vilib>:"Unflatten From JSON String.vi"("Type and Defaults"=w260, "error in (no error)"=w264, "JSON String"=w266) -> ("error out"=w267:errorcluster, "Variant"=w268:variant)  [unwired: 7 in]
                n97 = Variant To Data(error in=w267, type=w260, Variant=w268) -> (data=w265:T11, error out=w263:errorcluster)
                n98 = Unbundle By Name(w265) -> ("json.Method"=w262:string, "json.Seed"=w259:dbl)
                n99 = local write "范围_RandomNumber"(w259) -> ()
              }
              frame "CalculateNumber" {
                n100 = Unbundle By Name(w279) -> ("CalculateNumber"=w278:T12)
                n101 = call <vilib>:"Unflatten From JSON String.vi"("Type and Defaults"=w278, "error in (no error)"=w282, "JSON String"=w284) -> ("error out"=w285:errorcluster, "Variant"=w286:variant)  [unwired: 7 in]
                n102 = Variant To Data(error in=w285, type=w278, Variant=w286) -> (data=w283:T12, error out=w281:errorcluster)
                n103 = Unbundle By Name(w283) -> ("json.Method"=w280:string, "json.Type"=w273:string, "json.NumxVar"=w271:string, "json.NumyVar"=w270:string, "json.Formula"=w269:string)
                n104 = property on="变量数量_CalculateNumber" class="Enum (strict)"() -> ("Strings []"=w274:string[])  [unwired: 2 in, 2 out]
                n105 = local write "数值X_CalculateNumber"(w271) -> ()
                n106 = local write "数值Y_CalculateNumber"(w270) -> ()
                n107 = local write "公式"(w269) -> ()
                n108 = Search 1D Array(1D array=w274, element=w273) -> (index of element=w277:i32)  [unwired: 1 in]
                n109 = Greater Or Equal To 0?(x=w277) -> (x >= 0?=w276:bool)
                n110 = Select(t=w277, s=w276, f=0) -> (s? t:f=w272:i32)
                n111 = property on="变量数量_CalculateNumber" class="Enum (strict)"("Value"=w272) -> ()  [unwired: 2 in, 2 out]
              }
              frame "CompareNumber" {
                n112 = Unbundle By Name(w296) -> ("CompareNumber"=w295:T13)
                n113 = call <vilib>:"Unflatten From JSON String.vi"("Type and Defaults"=w295, "error in (no error)"=w299, "JSON String"=w301) -> ("error out"=w302:errorcluster, "Variant"=w303:variant)  [unwired: 7 in]
                n114 = Variant To Data(error in=w302, type=w295, Variant=w303) -> (data=w300:T13, error out=w298:errorcluster)
                n115 = Unbundle By Name(w300) -> ("json.Method"=w297:string, "json.Type"=w291:string, "json.NumxVar"=w288:string, "json.NumyVar"=w287:string)
                n116 = local write "数值Y_CompareNumber"(w287) -> ()
                n117 = local write "数值X_CompareNumber"(w288) -> ()
                n118 = property on="比较类型__CompareNumber" class="Ring (strict)"() -> ("Strings []"=w290:string[])  [unwired: 2 in, 2 out]
                n119 = Search 1D Array(1D array=w290, element=w291) -> (index of element=w294:i32)  [unwired: 1 in]
                n120 = Greater Or Equal To 0?(x=w294) -> (x >= 0?=w293:bool)
                n121 = Select(t=w294, s=w293, f=0) -> (s? t:f=w289:i32)
                n122 = property on="比较类型__CompareNumber" class="Ring (strict)"("Value"=w289) -> ()  [unwired: 2 in, 2 out]
              }
              frame Default {
              }
            }
            n123 = property on="方法" class="Enum (strict)"() -> ("Strings []"=w238:string[])  [unwired: 2 in, 2 out]
            n124 = Search 1D Array(1D array=w238, element=w236) -> (index of element=w240:i32)  [unwired: 1 in]
            n125 = Greater Or Equal To 0?(x=w240) -> (x >= 0?=w239:bool)
            n126 = Select(t=w240, s=w239, f=0) -> (s? t:f=w235:i32)
            n127 = local write "ArrayType"(w235) -> ()
            n128 = property on="方法" class="Enum (strict)"("Value"=w235) -> ()  [unwired: 2 in, 2 out]
          }
          frame True {
          }
        }
        n129 = call <vilib>:"Add State(s) to Queue__JKI_lib_State_Machine.vi"("State(s) in (\"\")"=w234) -> ("States Out"=w233:string)  [unwired: 14 in]
      }
      frame "Parameter: Combin Parameter" {
        n130 = property on="方法" class="Enum (strict)"() -> ("RingText.Text"=w307:string)  [unwired: 2 in, 2 out]
        n131 = case shown="\"InitialNumber\"" w307 {
          selector: w307 -> [_ w316 w326 w338 w349]
          tunnel: w310 -> [_ w323 w332 w344 w355]
          tunnel: [_ w321 w330 w342 w353] -> w306
          tunnel: [w314 w315 w325 w337 w348] -> w309
          tunnel: w308 -> [w314 w319 w328 w340 w351]
          frame Default {
          }
          frame "InitialNumber" {
            n132 = Unbundle By Name(w323) -> ("NumberClusters.InitialNumber"=w322:T10)
            n133 = local read "数值_InitialNumber"() -> (w318:dbl)
            n134 = Bundle By Name(cluster=w322, "json.Method"=w316, "json.InitialNum"=w318) -> (w317:T10)
            n135 = call <vilib>:"Flatten To JSON String.vi"("Multiline (T)"=TRUE, "error in (no error)"=w319, "Variant"=w317) -> ("error out"=w315:errorcluster, "JSON String"=w321:string)  [unwired: 7 in]
          }
          frame "RandomNumber" {
            n136 = Unbundle By Name(w332) -> ("NumberClusters.RandomNumber"=w331:T11)
            n137 = local read "范围_RandomNumber"() -> (w324:dbl)
            n138 = Bundle By Name(cluster=w331, "json.Method"=w326, "json.Seed"=w324) -> (w327:T11)
            n139 = call <vilib>:"Flatten To JSON String.vi"("Multiline (T)"=TRUE, "error in (no error)"=w328, "Variant"=w327) -> ("error out"=w325:errorcluster, "JSON String"=w330:string)  [unwired: 7 in]
          }
          frame "CalculateNumber" {
            n140 = local read "数值X_CalculateNumber"() -> (w335:string)
            n141 = property on="变量数量_CalculateNumber" class="Enum (strict)"() -> ("RingText.Text"=w336:string)  [unwired: 2 in, 2 out]
            n142 = local read "数值Y_CalculateNumber"() -> (w334:string)
            n143 = local read "公式"() -> (w333:string)
            n144 = Unbundle By Name(w344) -> ("NumberClusters.CalculateNumber"=w343:T12)
            n145 = Bundle By Name(cluster=w343, "json.Method"=w338, "json.Type"=w336, "json.NumxVar"=w335, "json.NumyVar"=w334, "json.Formula"=w333) -> (w339:T12)
            n146 = call <vilib>:"Flatten To JSON String.vi"("Multiline (T)"=TRUE, "error in (no error)"=w340, "Variant"=w339) -> ("error out"=w337:errorcluster, "JSON String"=w342:string)  [unwired: 7 in]
          }
          frame "CompareNumber" {
            n147 = local read "数值X_CompareNumber"() -> (w346:string)
            n148 = local read "数值Y_CompareNumber"() -> (w345:string)
            n149 = property on="比较类型__CompareNumber" class="Ring (strict)"() -> ("RingText.Text"=w347:string)  [unwired: 2 in, 2 out]
            n150 = Unbundle By Name(w355) -> ("NumberClusters.CompareNumber"=w354:T13)
            n151 = Bundle By Name(cluster=w354, "json.Method"=w349, "json.Type"=w347, "json.NumxVar"=w346, "json.NumyVar"=w345) -> (w350:T13)
            n152 = call <vilib>:"Flatten To JSON String.vi"("Multiline (T)"=TRUE, "error in (no error)"=w351, "Variant"=w350) -> ("error out"=w348:errorcluster, "JSON String"=w353:string)  [unwired: 7 in]
          }
        }
        n153 = Bundle By Name(cluster=w310, "Synchronize.Echo.JsonOut"=w306) -> (w311:T7)
        n154 = call <vilib>:"Add State(s) to Queue__JKI_lib_State_Machine.vi"("State(s) in (\"\")"=w313) -> ("States Out"=w312:string)  [unwired: 14 in]
      }
      frame "---------- Sync ----------" {
        n155 = call <vilib>:"Add State(s) to Queue__JKI_lib_State_Machine.vi"("State(s) in (\"\")"=w359) -> ("States Out"=w358:string)  [unwired: 14 in]
      }
      frame "Sync: Obtain CMD Queue" {
        # "这里由平台输入"
        n156 = Unbundle By Name(w361) -> ("Synchronize.EnqueueData"=w360:T14)
        n157 = Obtain Queue(name (unnamed)="VIId", element data type=w360, error in (no error)=w366) -> (queue out=w362:refnum<queue>, error out=w365:errorcluster)  [unwired: 2 in, 1 out]
        n158 = Bundle By Name(cluster=w361, "Synchronize.Queue"=w362) -> (w363:T7)
        n159 = call <vilib>:"Add State(s) to Queue__JKI_lib_State_Machine.vi"("State(s) in (\"\")"=w368) -> ("States Out"=w367:string)  [unwired: 14 in]
      }
      frame "Sync: Dequeue CMD" {
        n160 = Unbundle By Name(w381) -> ("Synchronize.Queue"=w378:refnum<queue>, "Synchronize.Communicate"=w369:T15)
        n161 = Dequeue Element(queue=w378, timeout in ms (-1)=10, error in (no error)=w379) -> (queue out=w377:refnum<queue>, element=w375:T14, timed out?=w376:bool, error out=w371:errorcluster)
        n162 = Bundle By Name(cluster=w381, "Synchronize.Queue"=w377, "Synchronize.EnqueueData"=w375) -> (w373:T7)
        n163 = case shown="False" w376 {
          tunnel: w375 -> [w392 _]
          tunnel: [w390 _] -> w374
          tunnel: w373 -> [w389 w421]
          tunnel: [w388 w421] -> w372
          tunnel: w371 -> [w386 w420]
          tunnel: [w385 w420] -> w370
          tunnel: w369 -> [w384 _]
          frame False {
            n164 = Unbundle By Name(w392) -> ("Action"=w391:T16, "Data"=w387:variant)
            n165 = case shown="\"Query\"" w391 {
              tunnel: ["Sync: Send ECHO" "UI: Initialize VarList\nSync: Send ECHO" _ "Sync: Send ECHO\nMacro: Exit" "Parameter: Combin Parameter\nSync: Send ECHO" "Parameter: Parse Parameter\nSync: Send ECHO"] -> w390
              tunnel: w389 -> [w395 w400 w404 w407 w412 w417]
              tunnel: [w394 w399 w404 w406 w411 w416] -> w388
              tunnel: w387 -> [_ _ _ _ _ _]
              tunnel: w386 -> [w396 w401 w403 w408 w413 w418]
              tunnel: [w396 w401 w403 w408 w413 w418] -> w385
              tunnel: w384 -> [_ _ _ _ _ _]
              frame "Create" {
                n166 = Bundle By Name(cluster=w395, "Synchronize.Echo.Status"="Create Success") -> (w394:T7)
              }
              frame "UpdateVariable" {
                n167 = Bundle By Name(cluster=w400, "Synchronize.Echo.Status"="UpdateVariable Success") -> (w399:T7)
              }
              frame Default {
              }
              frame "Close" {
                n168 = Bundle By Name(cluster=w407, "Synchronize.Echo.Status"="Close Success") -> (w406:T7)
              }
              frame "Query" {
                n169 = Bundle By Name(cluster=w412, "Synchronize.Echo.Status"="Query Success") -> (w411:T7)
              }
              frame "Revert" {
                n170 = Bundle By Name(cluster=w417, "Synchronize.Echo.Status"="Revert Success") -> (w416:T7)
              }
            }
          }
          frame True {
          }
        }
        n171 = call <vilib>:"Add State(s) to Queue__JKI_lib_State_Machine.vi"("State(s) in Front (\"\")"=w374, "State(s) in (\"\")"=w383) -> ("States Out"=w382:string)  [unwired: 13 in]
      }
      frame "Sync: Release CMD Queue" {
        n172 = Unbundle By Name(w424) -> ("Synchronize.Queue"=w425:refnum<queue>)
        n173 = Release Queue(queue=w425, error in (no error)=w423) -> (error out=w422:errorcluster)  [unwired: 1 in, 2 out]
        n174 = call <vilib>:"Add State(s) to Queue__JKI_lib_State_Machine.vi"("State(s) in (\"\")"=w427) -> ("States Out"=w426:string)  [unwired: 14 in]
      }
      frame "Sync: Send ECHO" {
        n175 = Unbundle By Name(w431) -> ("Synchronize.Communicate"=w428:T15, "Synchronize.EnqueueData.Data"=w440:variant, "Synchronize.Echo"=w432:T17)
        n176 = Variant To Data(error in=w430, type=w428, Variant=w440) -> (data=w433:T15, error out=w434:errorcluster)
        n177 = Unbundle By Name(w433) -> ("ID"=w437:string)
        n178 = Obtain Queue(name (unnamed)=w437, element data type=w432, error in (no error)=w434) -> (queue out=w436:refnum<queue>, error out=w438:errorcluster)  [unwired: 2 in, 1 out]
        n179 = Enqueue Element(queue=w436, element=w432, error in (no error)=w438) -> (queue out=w435:refnum<queue>, error out=w439:errorcluster)  [unwired: 1 in, 1 out]
        n180 = Release Queue(queue=w435, error in (no error)=w439) -> (error out=w429:errorcluster)  [unwired: 1 in, 2 out]
        n181 = call <vilib>:"Add State(s) to Queue__JKI_lib_State_Machine.vi"("State(s) in (\"\")"=w442) -> ("States Out"=w441:string)  [unwired: 14 in]
      }
    }
  }
  n182 = flat-sequence {
    frame #0 {
    }
  }
